vi "MecaOdometry_New.vi"(8 "Initial Pose2d":T5={"TRANSLATION"={"X"=0.0, "Y"=0.0}, "ROTATION"={"VALUE"=0.0, "COS"=1.0, "SIN"=0.0}} {"ROTATION"."SIN" format="%13.4f"; "ROTATION"."COS" format="%13.4f"; "ROTATION"."VALUE" format="%13.4f"; "TRANSLATION"."Y" format="%14.3f"; "TRANSLATION"."X" format="%14.3f"}, 9 "wheelPositions":T1 {"RearRight" format="%19.3f"; "RearLeft" format="%19.3f"; "FrontRight" format="%19.3f"; "FrontLeft" format="%19.3f"}, 10 "GyroOffset":T6 {"SIN" format="%13.4f"; "COS" format="%13.4f"; "VALUE" format="%13.4f"}, 11 "Mecanum Kinematics":T2={"FrontLeft"={"X"=0.0, "Y"=0.0}, "FrontRight"={"X"=0.0, "Y"=0.0}, "RearLeft"={"X"=0.0, "Y"=0.0}, "RearRight"={"X"=0.0, "Y"=0.0}, "InverseKinematics"=[[0.0, 1.0, -1.0, 0.0], [0.0, 1.0, 1.0, 0.0], [0.0, 1.0, 1.0, 0.0], [0.0, 1.0, -1.0, 0.0]], "ForwardKinematics"=[[0.0, 1.0, -1.0, 0.0], [0.0, 1.0, 1.0, 0.0], [0.0, 1.0, 1.0, 0.0], [0.0, 1.0, -1.0, 0.0]], "PrevCoR"={"X"=0.0, "Y"=0.0}} {"PrevCoR"."Y" format="%14.3f"; "PrevCoR"."X" format="%14.3f"; "RearRight"."Y" format="%14.3f"; "RearRight"."X" format="%14.3f"; "RearLeft"."Y" format="%14.3f"; "RearLeft"."X" format="%14.3f"; "FrontRight"."Y" format="%14.3f"; "FrontRight"."X" format="%14.3f"; "FrontLeft"."Y" format="%14.3f"; "FrontLeft"."X" format="%14.3f"}) -> (3 "MECA_DRIVE_ODOMETRY":T7={"POSE"={"TRANSLATION"={"X"=0.0, "Y"=0.0}, "ROTATION"={"VALUE"=0.0, "COS"=1.0, "SIN"=0.0}}, "GyroOffset"={"VALUE"=0.0, "COS"=0.0, "SIN"=0.0}, "PreviousAngle"={"VALUE"=0.0, "COS"=0.0, "SIN"=0.0}, "Kinematics"={"FrontLeft"={"X"=0.0, "Y"=0.0}, "FrontRight"={"X"=0.0, "Y"=0.0}, "RearLeft"={"X"=0.0, "Y"=0.0}, "RearRight"={"X"=0.0, "Y"=0.0}, "InverseKinematics"=[[0.0, 1.0, -1.0, 0.0], [0.0, 1.0, 1.0, 0.0], [0.0, 1.0, 1.0, 0.0], [0.0, 1.0, -1.0, 0.0]], "ForwardKinematics"=[[0.0, 1.0, -1.0, 0.0], [0.0, 1.0, 1.0, 0.0], [0.0, 1.0, 1.0, 0.0], [0.0, 1.0, -1.0, 0.0]], "PrevCoR"={"X"=0.0, "Y"=0.0}}, "PreviousWheelPositions"={"FrontLeft"=0.0, "FrontRight"=0.0, "RearLeft"=0.0, "RearRight"=0.0, "P"=FALSE}} {"PreviousWheelPositions"."RearRight" format="%19.3f"; "PreviousWheelPositions"."RearLeft" format="%19.3f"; "PreviousWheelPositions"."FrontRight" format="%19.3f"; "PreviousWheelPositions"."FrontLeft" format="%19.3f"; "Kinematics"."PrevCoR"."Y" format="%14.3f"; "Kinematics"."PrevCoR"."X" format="%14.3f"; "Kinematics"."RearRight"."Y" format="%14.3f"; "Kinematics"."RearRight"."X" format="%14.3f"; "Kinematics"."RearLeft"."Y" format="%14.3f"; "Kinematics"."RearLeft"."X" format="%14.3f"; "Kinematics"."FrontRight"."Y" format="%14.3f"; "Kinematics"."FrontRight"."X" format="%14.3f"; "Kinematics"."FrontLeft"."Y" format="%14.3f"; "Kinematics"."FrontLeft"."X" format="%14.3f"; "PreviousAngle"."SIN" format="%13.4f"; "PreviousAngle"."COS" format="%13.4f"; "PreviousAngle"."VALUE" format="%13.4f"; "GyroOffset"."SIN" format="%13.4f"; "GyroOffset"."COS" format="%13.4f"; "GyroOffset"."VALUE" format="%13.4f"; "POSE"."ROTATION"."SIN" format="%13.4f"; "POSE"."ROTATION"."COS" format="%13.4f"; "POSE"."ROTATION"."VALUE" format="%13.4f"; "POSE"."TRANSLATION"."Y" format="%14.3f"; "POSE"."TRANSLATION"."X" format="%14.3f"})   [LabVIEW 2019, in "Trajectory_Library.lvlib"]
doc: "Constructs a MecanumDriveOdometry cluster data structure\n\nSubVIs for mecanum drive odometry. Odometry allows you to track the robot's position on the field over a course of a match using readings from your mecanum wheel encoders.\n\nTeams can use odometry during the autonomous period for complex tasks like path following. Furthermore, odometry can be used for latency compensation when using computer-vision systems.\n\nParameters:\n - Mecanum Kinematics -- The mechanum kinematics data cluster for this drive\n - GyroOffset - The angle reported by the gyroscope. (Rotation)\n - wheelPositions -- The distances driven by each wheel.\n - initialPose - The starting position of the robot on the field. (Pose - Meters)\n\nReturns:\n - MecaDriveOdomentry - Data structure"
uses:
  Trajectory_Library.lvlib
  TypeDef/TRANSLATION2D.ctl
  TypeDef/ROTATION2D.ctl
  TypeDef/POSE2D.ctl
  TypeDef/MECA_DRIVE_ODOMETRY.ctl
  <vilib>/Rock Robotics/SystemInterfaces/NetworkCommunication/NetComm_UsageReport_ResourceType.ctl
  Util_LibraryGlobals.vi
  <vilib>/Analysis/Matrix/Datatypes/RealMatrix.ctl
  <vilib>/Analysis/Matrix/NI_Matrix.lvlib
  TypeDef/MECA_DRIVE_KINEMATICS.ctl
  TypeDef/MECA_WHEEL_POSITIONS.ctl
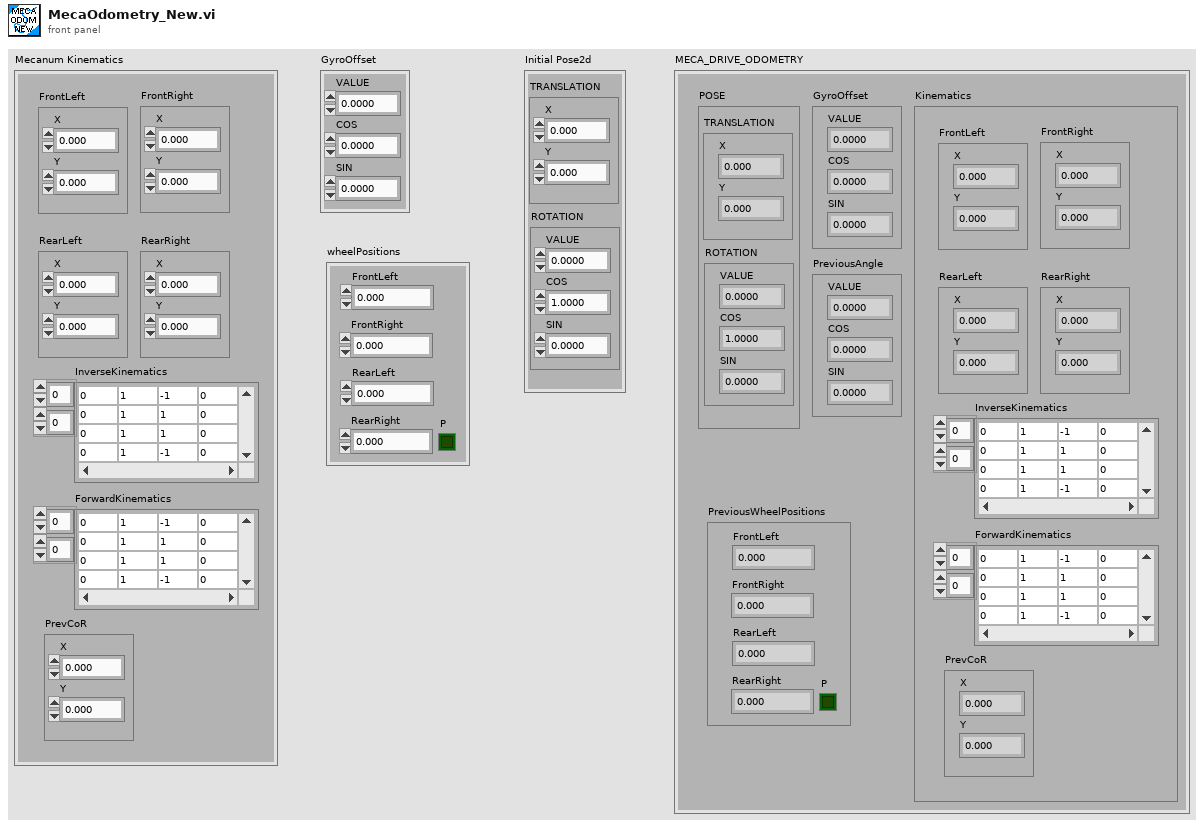
[diagram p1: front panel]
types:
  T1 = typedef "Trajectory_Library.lvlib/MECA_WHEEL_POSITIONS.ctl" = cluster{"FrontLeft":dbl, "FrontRight":dbl, "RearLeft":dbl, "RearRight":dbl, "P":bool}
  T2 = typedef "Trajectory_Library.lvlib/MECA_DRIVE_KINEMATICS.ctl" = cluster{"FrontLeft":T3, "FrontRight":T3, "RearLeft":T3, "RearRight":T3, "InverseKinematics":T4, "ForwardKinematics":T4, "PrevCoR":T3}
  T3 = typedef "Trajectory_Library.lvlib/TRANSLATION2D.ctl" = cluster{"X":dbl, "Y":dbl}
  T4 = typedef "NI_Matrix.lvlib/RealMatrix.ctl" = dbl[][]
  T5 = typedef "Trajectory_Library.lvlib/POSE2D.ctl" = cluster{"TRANSLATION":T3, "ROTATION":T6}
  T6 = typedef "Trajectory_Library.lvlib/ROTATION2D.ctl" = cluster{"VALUE":dbl, "COS":dbl, "SIN":dbl}
  T7 = typedef "Trajectory_Library.lvlib/MECA_DRIVE_ODOMETRY.ctl" = cluster{"POSE":T5, "GyroOffset":T6, "PreviousAngle":T6, "Kinematics":T2, "PreviousWheelPositions":T1}
  T8 = typedef "NetComm_UsageReport_ResourceType.ctl" = enum8{"Controller", "Module", "Language", "CANPlugin", "Accelerometer", "ADXL345", "AnalogChannel", "AnalogTrigger", "AnalogTriggerOutput", "CANJaguar", "Compressor", "Counter", "Dashboard", "DigitalInput", "DigitalOutput", "DriverStationCIO", "DriverStationEIO", "DriverStationLCD", "Encoder", "GearTooth", "Gyro", "I2C", "Framework", "Jaguar", "Joystick", "Kinect", "KinectStick", "PIDController", "Preferences", "PWM", "Relay", "RobotDrive", "SerialPort", "Servo", "Solenoid", "SPI", "Task", "Ultrasonic", "Victor", "Button", "Command", "AxisCamera", "PCVideoServer", "SmartDashboard", "Talon", "HiTechnicColorSensor", "HiTechnicAccel", "HiTechnicCompass", "SRF08", "AnalogOutput", "Victor SP", "Talon SRX", "CAN Talon SRX", "ADXL362 Accel", "ADXRS450 Gyro", "Rev SPARK", "Mindsensors SD540", "Digital Filter", "ADIS16448", "PDP", "PCM", "PigeonIMU", "Nidec Brushless", "CTRE CANifier", "CTRE TalonFX", "CTRE Future 1", "CTRE Future 2", "CTRE Future 3", "CTRE Future 4", "CTRE Future 5", "CTRE Future 6", "Linear Filter", "Xbox Controller", "USB Camera", "NavX", "Pixy", "Pixy2", "ScanseSweep", "Shuffleboard", "CAN", "Digilent DMC60", "PWM Victor SPX", "Rev SPARK MAX PWM", "Rev SPARK MAX CAN", "ADIS16470", "PIDController2", "ProfiledPIDController", "Kinematics", "Odometry", "Units", "Trapezoid Profile", "DutyCycle", "Addressable LEDs", "Fusion Venom"}
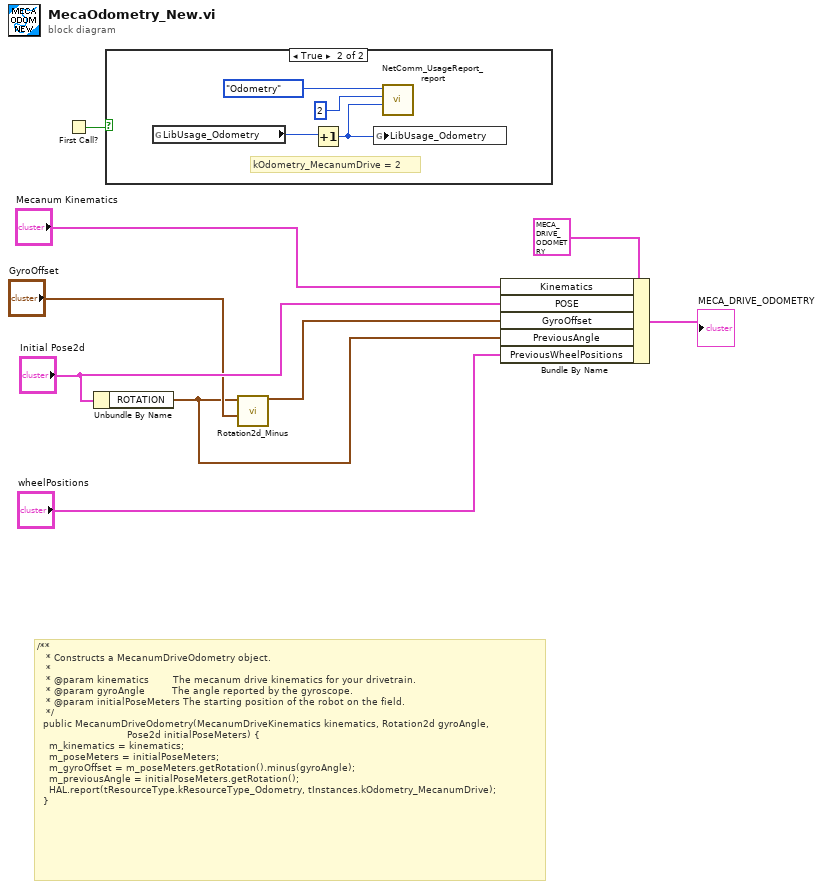
[diagram p0: block diagram]
diagram:
  # "/**\n   * Constructs a MecanumDriveOdometry object.\n   *\n   * @param kinematics        The mecanum drive kinematics for your drivetrain.\n   * @param gyroAngle         The angle reported by the gyroscope.\n   * @param initialPoseMeters The starting position of the robot on the field.\n   */\n  public MecanumDriveOdometry(MecanumDriveKinematics kinematics, Rotation2d gyroAngle,\n                              Pose2d initialPoseMeters) {\n    m_kinematics = kinematics;\n    m_poseMeters = initialPoseMeters;\n    m_gyroOffset = m_poseMeters.getRotation().minus(gyroAngle);\n    m_previousAngle = initialPoseMeters.getRotation();\n    HAL.report(tResourceType.kResourceType_Odometry, tInstances.kOdometry_MecanumDrive);\n  }"
  n1 = First Call?() -> (First Call?: T/F=w3:bool)
  n2 = Unbundle By Name("Initial Pose2d") -> ("ROTATION"=w4:T6)
  n3 = case shown="True" w3 {
    frame False {
    }
    frame True {
      # "kOdometry_MecanumDrive = 2"
      n4 = global read "Util_LibraryGlobals.vi" "LibUsage_Odometry"() -> (w12:i32)
      n5 = Increment(x=w12) -> (x+1=w11:i32)
      n6 = global write "Util_LibraryGlobals.vi" "LibUsage_Odometry"(w11) -> ()
      n7 = call <vilib>:"NetComm_UsageReport_report.vi"("Context"=w11, "Instance Number"=u8 2, "Resource Type"=NetComm_UsageReport_ResourceType."Odometry") -> ()  [unwired: 9 in]
    }
  }
  n8 = call "Rotation2d_Minus.vi"("other ROTATION"="GyroOffset", "in ROTATION"=w4) -> ("out ROTATION"=w5:T6)  [unwired: 9 in]
  n9 = Bundle By Name(cluster=T7 {"POSE"={"TRANSLATION"={"X"=0.0, "Y"=0.0}, "ROTATION"={"VALUE"=0.0, "COS"=1.0, "SIN"=0.0}}, "GyroOffset"={"VALUE"=0.0, "COS"=0.0, "SIN"=0.0}, "PreviousAngle"={"VALUE"=0.0, "COS"=0.0, "SIN"=0.0}, "Kinematics"={"FrontLeft"={"X"=0.0, "Y"=0.0}, "FrontRight"={"X"=0.0, "Y"=0.0}, "RearLeft"={"X"=0.0, "Y"=0.0}, "RearRight"={"X"=0.0, "Y"=0.0}, "InverseKinematics"=[[0.0, 1.0, -1.0, 0.0], [0.0, 1.0, 1.0, 0.0], [0.0, 1.0, 1.0, 0.0], [0.0, 1.0, -1.0, 0.0]], "ForwardKinematics"=[[0.0, 1.0, -1.0, 0.0], [0.0, 1.0, 1.0, 0.0], [0.0, 1.0, 1.0, 0.0], [0.0, 1.0, -1.0, 0.0]], "PrevCoR"={"X"=0.0, "Y"=0.0}}, "PreviousWheelPositions"={"FrontLeft"=0.0, "FrontRight"=0.0, "RearLeft"=0.0, "RearRight"=0.0, "P"=FALSE}} ("MECA_DRIVE_ODOMETRY"), "Kinematics"="Mecanum Kinematics", "POSE"="Initial Pose2d", "GyroOffset"=w5, "PreviousAngle"=w4, "PreviousWheelPositions"="wheelPositions") -> (→"MECA_DRIVE_ODOMETRY":T7)
